vi "IG_Control.vi"(0 "Time Since Shot (s)":dbl=0.0001, 1 "After Shot Wait (s)":dbl, 2 "appended array":T2[](array[typedef]) {"CG2 Vac Level" format="%#_2e"; "CG1 Vac Level" format="%#_2e"; "IG Vac Level" format="%#_2e"}, 3 "IG Control In":bool, 4 "IG Select":bool, 5 "Charge Step":T1(ring)) -> (20 "IG1 Control Out":bool, 24 "IG2 Control Out":bool)   [LabVIEW 2009]
uses:
  VacuumControls.ctl
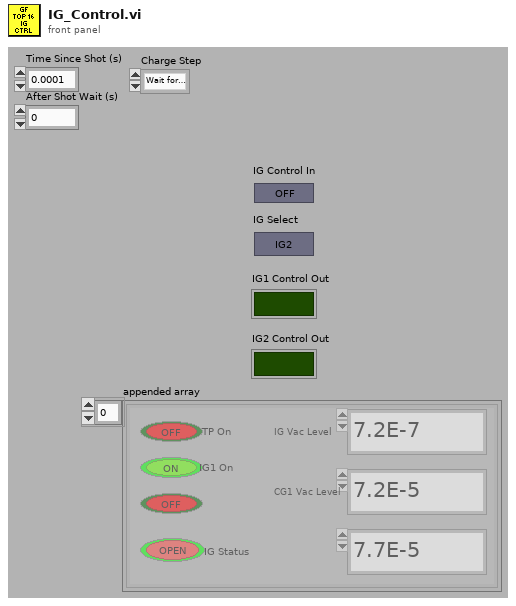
[diagram p1: front panel]
types:
  T1 = enum16{"Wait for Ready", "Prep for Charge", "Open Dump Relays", "Close Connect Relays", "Wait PS Delays", "Wait End of Charge", "Turn Off HV", "Open Connect Relays", "Charge Done"}
  T2 = typedef "VacuumControls.ctl" = cluster{"TP On":bool, "IG1 On":bool, "IG2On":bool, "IG Vac Level":dbl, "CG1 Vac Level":dbl, "CG2 Vac Level":dbl, "IG Status":bool}
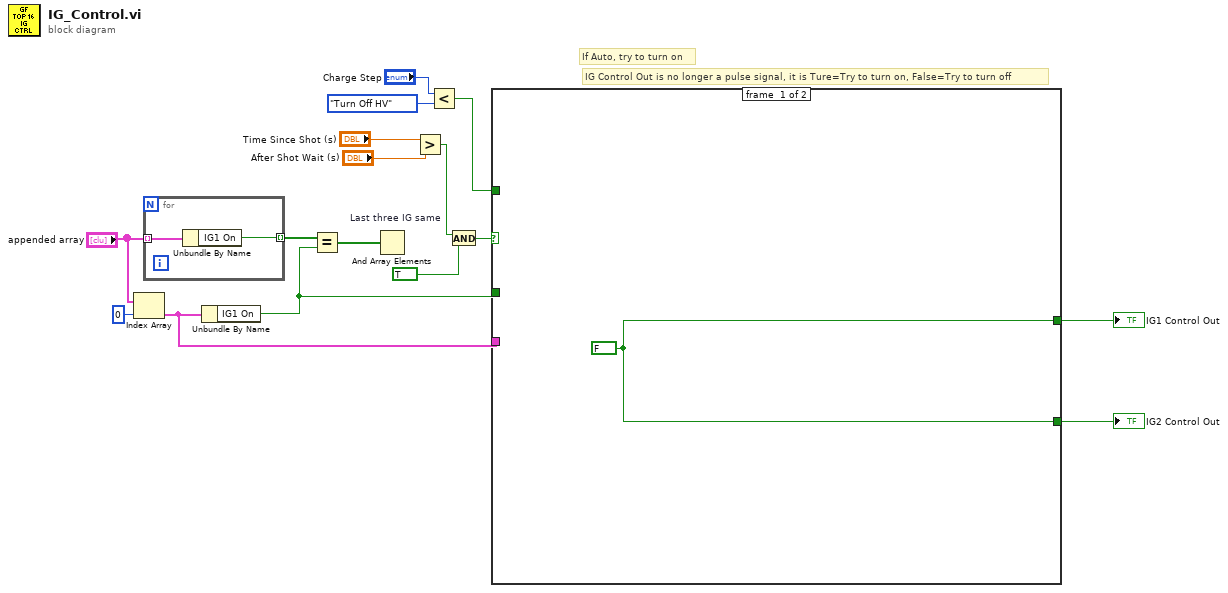
[diagram p0: block diagram]
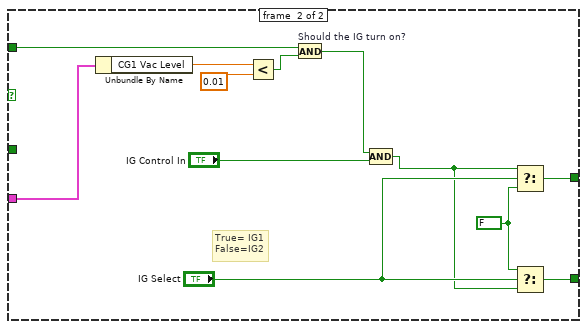
[diagram p2: hidden frame]
diagram:
  # "IG Control Out is no longer a pulse signal, it is Ture=Try to turn on, False=Try to turn off"
  # "If Auto, try to turn on"
  n1 = Index Array(array="appended array", index=0) -> (element=w12:T2)
  n2 = for {
    tunnel: "appended array" -> [w18] mode=indexing
    tunnel: [w17] -> w14 mode=indexing
    n3 = Unbundle By Name(w18) -> ("IG1 On"=w17:bool)
  }
  n4 = Unbundle By Name(w12) -> ("IG1 On"=w9:bool)
  n5 = Equal?(x=w14, y=w9) -> (x = y?=w13:bool[])
  n6 = And Array Elements "Last three IG same"(Boolean array=w13) -> ()  [unwired: 1 out]
  n7 = Greater?(x="Time Since Shot (s)", y="After Shot Wait (s)") -> (0:w5:bool)
  n8 = Less?(x="Charge Step", y=T1."Turn Off HV") -> (x < y?=w2:bool)
  n9 = And(x=w5, y=TRUE) -> (x .and. y?=w6:bool)
  n10 = case shown="True" w6 {
    tunnel: w12 -> [_ w31]
    tunnel: [w19 w30] -> w11
    tunnel: [w19 w29] -> w10
    tunnel: w9 -> [_ _]
    tunnel: w2 -> [_ w22]
    frame #0 {
      w19 = FALSE ("IG1 pulse")
    }
    frame #1 {
      w26 = FALSE
      # "True= IG1\nFalse=IG2"
      n11 = Unbundle By Name(w31) -> ("CG1 Vac Level"=w27:dbl)
      n12 = Less?(x=w27, y=0.01) -> (x < y?=w24:bool)
      n13 = And "Should the IG turn on?"(x=w22, y=w24) -> (x .and. y?=w23:bool)
      n14 = Compound Arithmetic op=AND(w23, "IG Control In") -> (w20:bool)
      n15 = Select(t=w20, s="IG Select", f=w26) -> (s? t:f=w30:bool)
      n16 = Select(t=w26, s="IG Select", f=w20) -> (s? t:f=w29:bool)
    }
  }
  "IG1 Control Out" <- w11
  "IG2 Control Out" <- w10
